vi "Filter scale.vi"(1 "Raw Photon Count":dbl, 2 "filter data":cluster{"Numeric":dbl, dbl}[](array[cluster]), 3 "Energy (J)":dbl) -> (0 "filter scaled count":dbl)   [LabVIEW 2019]
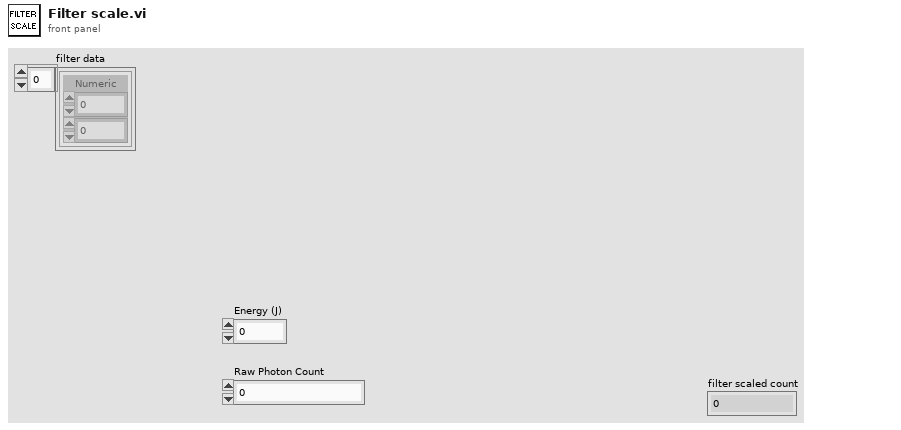
[diagram p1: front panel]
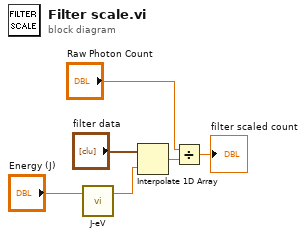
[diagram p0: block diagram]
diagram:
  n1 = call "J-eV.vi"("J"="Energy (J)") -> ("eV"=w2:dbl)  [unwired: 1 in, 1 out]
  n2 = Interpolate 1D Array(1:w2, 2:"filter data") -> (0:w4:dbl)
  n3 = Divide(x="Raw Photon Count", y=w4) -> (x/y=→"filter scaled count":dbl)
